vi "LV diagram.vi"() -> ()   [LabVIEW 2012]
panel:
  in  "vi path":path
  out "diagrams":string
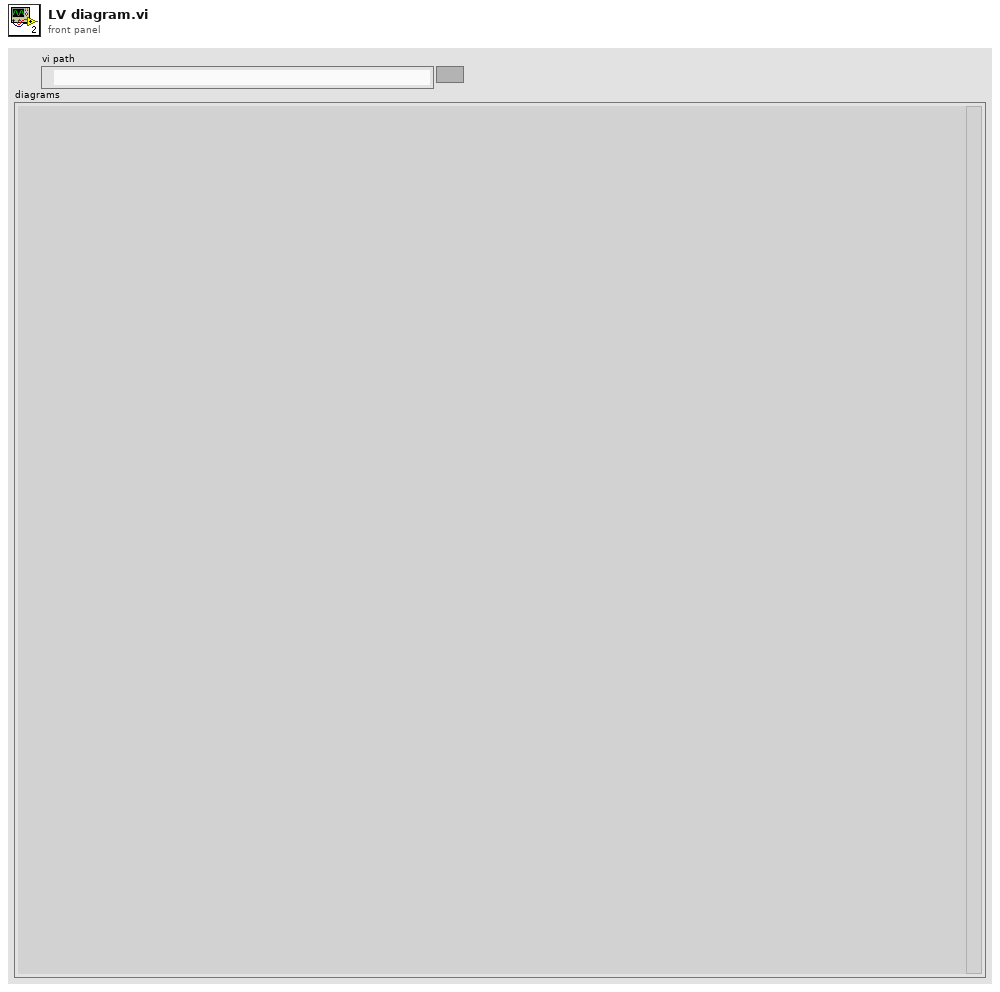
[diagram p1: front panel]
types:
  T1 = cluster{"index":i32, "index":i32, "Diagram":refnum<vi>}
  T2 = cluster{"index":i32, "index":i32, "Diagram":refnum<vi>}[]
  T3 = cluster{"UID":i32, "index":i32, "Diagram":refnum<vi>}[]
  T4 = cluster{"UID":i32, "index":i32, "Diagram":refnum<vi>}
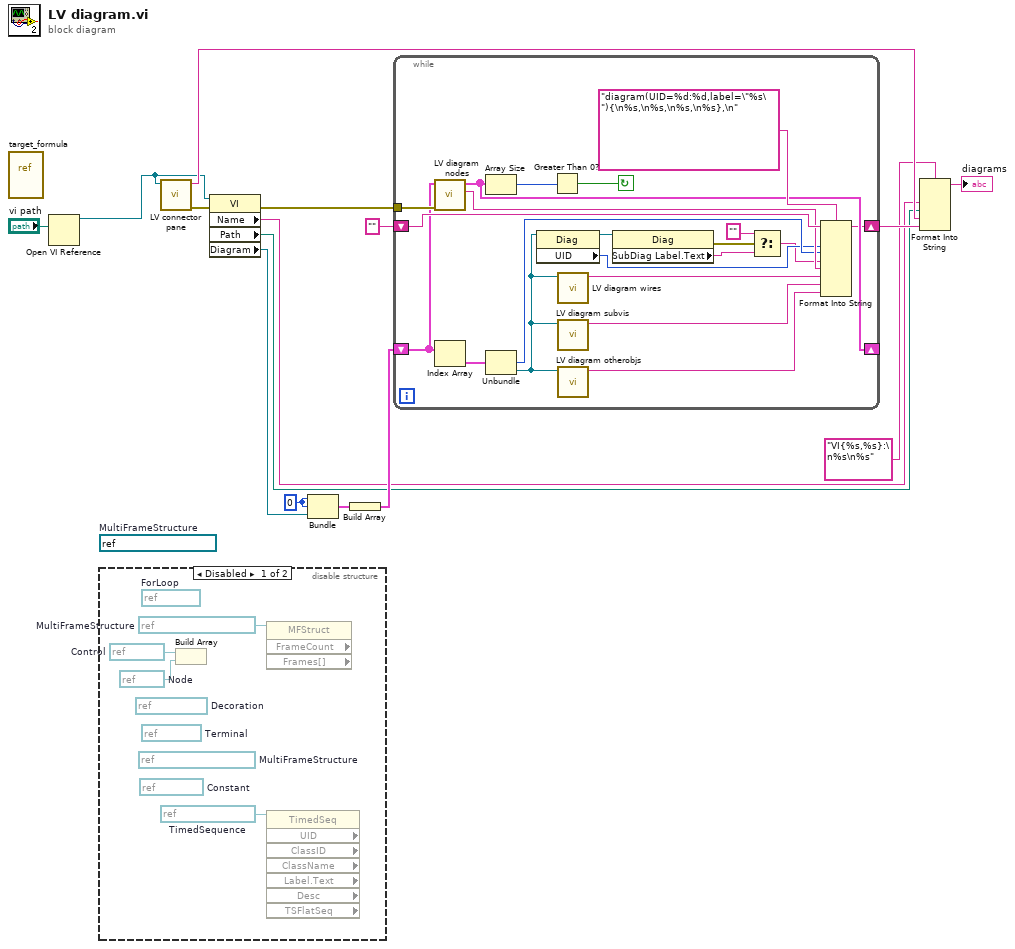
[diagram p0: block diagram]
diagram:
  (unwired) refnum<vi> refnum  # MultiFrameStructure
  w12 = 0 ("index")
  n1 = vi-ref "target_formula.vi"() -> ()  [unwired: 1 out]
  n2 = Open VI Reference(vi path="vi path") -> (vi reference=w2:refnum<vi>)  [unwired: 5 in, 1 out]
  n3 = disable-structure shown="Disabled" {
    frame Disabled {
      w16 = refnum<vi> refnum  # MultiFrameStructure
      w17 = refnum<vi> refnum  # TimedSequence
      (unwired) refnum<vi> refnum  # MultiFrameStructure
      (unwired) refnum<vi> refnum  # Terminal
      w18 = refnum<vi> refnum  # Node
      (unwired) refnum<vi> refnum  # Decoration
      w19 = refnum<vi> refnum  # Control
      (unwired) refnum<vi> refnum  # Constant
      (unwired) refnum<vi> refnum  # ForLoop
      n4 = Build Array(w19, w18) -> ()  [unwired: 1 out]
      n5 = property class="MFStruct" props=["FrameCount", "Frames[]"](reference=w16) -> ()  [unwired: 1 in, 4 out]
      n6 = property class="TimedSeq" props=["UID", "ClassID", "ClassName", "Label", "Text", "Desc", "TSFlatSeq"](reference=w17) -> ()  [unwired: 1 in, 8 out]
    }
    frame Enabled {
    }
  }
  n7 = call "LV connector pane.vi"("reference"=w2) -> ("error out"=w6:errorcluster, "conpane"=w10:string)  [unwired: 9 in]
  n8 = property class="VI"(reference=w2, error in=w6) -> (error out=w15:errorcluster, "Name"=w4:string, "Path"=w3:path, "Diagram"=w5:refnum<vi>)  [unwired: 1 out]
  n9 = Bundle("index"=w12, "index"=w12, "Diagram"=w5) -> (w13:T1)  [unwired: 1 in]
  n10 = Build Array(w13) -> (w14:T2)
  n11 = while {
    tunnel: w15 -> [w40]
    shift-right: [w32] -> w9
    shift-left: "" -> [w38]
    shift-right: [w35] -> _
    shift-left: w14 -> [w30]
    stop <- w36 continue-if-true
    n12 = call "LV diagram nodes.vi"("error in (no error)"=w40, "diagrams in"=w30) -> ("diagram desc."=w34:string, "diagrams out"=w35:T3)  [unwired: 8 in]
    n13 = Index Array(array=w30) -> (element=w31:T4)  [unwired: 1 in]
    n14 = Array Size(array=w35) -> (size(s)=w37:i32)
    n15 = Unbundle(w31) -> ("index"=w26:i32, "Diagram"=w27:refnum<vi>)  [unwired: 1 out]
    n16 = property class="Diag"(reference=w27) -> (reference out=w20:refnum<vi>, "UID"=w25:i32)  [unwired: 1 in, 1 out]
    n17 = Greater Than 0?(x=w37) -> (x > 0?=w36:bool)
    n18 = call "LV diagram wires.vi"("reference"=w27) -> ("wiring"=w33:string)  [unwired: 9 in, 1 out]
    n19 = call "LV diagram subvis.vi"("reference"=w27) -> ("sUBvIS"=w29:string)  [unwired: 10 in]
    n20 = call "LV diagram otherobjs.vi"("reference"=w27) -> ("String"=w28:string)  [unwired: 10 in]
    n21 = property class="Diag"(reference=w20) -> (error out=w23:errorcluster, "SubDiag Label.Text"=w24:string)  [unwired: 1 in, 1 out]
    n22 = Select(t="", s=w23, f=w24) -> (s? t:f=w21:string)
    n23 = Format Into String(format string="diagram(UID=%d:%d,label=\"%s\"){\n%s,\n%s,\n%s,\n%s},\n", initial string=w38, w25, w26, w21, w34, w33, w29, w28) -> (resulting string=w32:string)  [unwired: 1 in, 1 out]
  }
  n24 = Format Into String(format string="VI{%s,%s}:\n%s\n%s", w4, w3, w10, w9) -> (resulting string=→"diagrams":string)  [unwired: 2 in, 1 out]
